vi "Func-엑셀 데이터를 그래프로 출력.vi"() -> ()   [LabVIEW 2015] (continued)
-4.925\n-18.3\t-18.32\t-4.927\n-18.3\t-18.32\t-4.934\n-18.3\t-18.32\t-4.936\n-18.3\t-18.32\t-4.944\n-18.3\t-18.32\t-4.95\n-18.3\t-18.32\t-4.957\n-18.3\t-18.32\t-4.965\n-18.3\t-18.32\t-4.972\n-18.3\t-18.32\t-4.976\n-18.3\t-18.32\t-4.977\n-18.3\t-18.32\t-4.984\n-18.3\t-18.32\t-4.99\n-18.3\t-18.32\t-4.997\n-18.3\t-18.32\t-5.002\n-18.3\t-18.32\t-5.007\n-18.3\t-18.32\t-5.013\n-18.3\t-18.32\t-5.02\n-18.3\t-18.32\t-5.023\n-18.3\t-18.32\t-5.024\n-18.3\t-18.32\t-5.031\n-18.3\t-18.32\t-5.036\n-18.3\t-18.32\t-5.041\n-18.3\t-18.32\t-5.047\n-18.3\t-18.32\t-5.053\n-18.3\t-18.32\t-5.061\n-18.3\t-18.32\t-5.069\n-18.3\t-18.32\t-5.075\n-18.3\t-18.32\t-5.08\n-18.3\t-18.32\t-5.085\n-18.3\t-18.32\t-5.091\n-18.3\t-18.32\t-5.092\n-18.3\t-18.32\t-5.099\n-18.3\t-18.32\t-5.105\n-18.3\t-18.32\t-5.109\n-18.3\t-18.32\t-5.117\n-18.3\t-18.32\t-5.122\n-18.3\t-18.32\t-5.13\n-18.3\t-18.32\t-5.134\n-18.3\t-18.32\t-5.137\n-18.3\t-18.32\t-5.142\n-18.3\t-18.32\t-5.146\n-18.3\t-18.32\t-5.15\n-18.3\t-18.32\t-5.152\n-18.3\t-18.32\t-5.16\n-18.3\t-18.32\t-5.164\n-18.3\t-18.32\t-5.166\n-18.3\t-18.32\t-5.177\n-18.3\t-18.32\t-5.183\n-18.3\t-18.32\t-5.187\n-18.3\t-18.32\t-5.19\n-18.3\t-18.31\t-5.196\n-18.3\t-18.31\t-5.202\n-18.3\t-18.31\t-5.205\n-18.3\t-18.31\t-5.209\n-18.3\t-18.31\t-5.214\n-18.3\t-18.31\t-5.219\n-18.3\t-18.31\t-5.223\n-18.3\t-18.31\t-5.225\n-18.3\t-18.31\t-5.231\n-18.3\t-18.31\t-5.235\n-18.3\t-18.31\t-5.24\n-18.3\t-18.31\t-5.25\n-18.3\t-18.31\t-5.254\n-18.3\t-18.31\t-5.262\n-18.3\t-18.31\t-5.269\n-18.3\t-18.31\t-5.274\n-18.3\t-18.31\t-5.279\n-18.3\t-18.31\t-5.28\n-18.3\t-18.31\t-5.287\n-18.3\t-18.31\t-5.291\n-18.3\t-18.31\t-5.298\n-18.3\t-18.31\t-5.302\n-18.3\t-18.31\t-5.305\n-18.3\t-18.31\t-5.312\n-18.3\t-18.31\t-5.312\n-18.3\t-18.31\t-5.318\n-18.3\t-18.31\t-5.323\n-18.3\t-18.31\t-5.328\n-18.3\t-18.31\t-5.334\n-18.3\t-18.31\t-5.346\n-18.3\t-18.31\t-5.353\n-18.3\t-18.31\t-5.354\n-18.3\t-18.31\t-5.36\n-18.3\t-18.31\t-5.363\n-18.3\t-18.31\t-5.363\n-18.3\t-18.31\t-5.367\n-18.3\t-18.31\t-5.372\n-18.3\t-18.31\t-5.378\n-18.3\t-18.31\t-5.384\n-18.3\t-18.31\t-5.391\n-18.3\t-18.31\t-5.398\n-18.3\t-18.31\t-5.402\n-18.3\t-18.31\t-5.407\n-18.3\t-18.31\t-5.411\n-18.3\t-18.31\t-5.416\n-18.3\t-18.31\t-5.418\n-18.3\t-18.31\t-5.423\n-18.3\t-18.31\t-5.427\n-18.3\t-18.31\t-5.43\n-18.3\t-18.31\t-5.437\n-18.3\t-18.31\t-5.442\n-18.3\t-18.31\t-5.447\n-18.3\t-18.31\t-5.451\n-18.3\t-18.31\t-5.459\n-18.3\t-18.31\t-5.461\n-18.3\t-18.31\t-5.463\n-18.3\t-18.31\t-5.469\n-18.3\t-18.31\t-5.473\n-18.3\t-18.31\t-5.48\n-18.3\t-18.31\t-5.485\n-18.3\t-18.31\t-5.489\n-18.3\t-18.31\t-5.495\n-18.3\t-18.31\t-5.504\n-18.3\t-18.31\t-5.509\n-18.3\t-18.31\t-5.511\n-18.3\t-18.31\t-5.516\n-18.3\t-18.31\t-5.519\n-18.3\t-18.29\t-5.52\n-18.3\t-18.29\t-5.523\n-18.3\t-18.29\t-5.529\n-18.3\t-18.29\t-5.533\n-18.3\t-18.29\t-5.54\n-18.3\t-18.29\t-5.546\n-18.3\t-18.29\t-5.555\n-18.3\t-18.29\t-5.56\n-18.3\t-18.29\t-5.563\n-18.3\t-18.29\t-5.564\n-18.3\t-18.29\t-5.571\n-18.3\t-18.29\t-5.575\n-18.3\t-18.29\t-5.576\n-18.3\t-18.29\t-5.582\n-18.3\t-18.29\t-5.584\n-18.3\t-18.29\t-5.591\n-18.3\t-18.29\t-5.593\n-18.3\t-18.29\t-5.596\n-18.3\t-18.29\t-5.602\n-18.3\t-18.29\t-5.606\n-18.3\t-18.29\t-5.61\n-18.3\t-18.29\t-5.614\n-18.3\t-18.29\t-5.62\n-18.3\t-18.29\t-5.626\n-18.3\t-18.29\t-5.63\n-18.3\t-18.29\t-5.639\n-18.3\t-18.29\t-5.645\n-18.3\t-18.29\t-5.647\n-18.3\t-18.29\t-5.654\n-18.3\t-18.29\t-5.658\n-18.3\t-18.29\t-5.66\n-18.3\t-18.29\t-5.661\n-18.3\t-18.29\t-5.664\n-18.3\t-18.29\t-5.668\n-18.3\t-18.29\t-5.673\n-18.3\t-18.29\t-5.675\n-18.3\t-18.29\t-5.684\n-18.3\t-18.29\t-5.69\n-18.3\t-18.29\t-5.689\n-18.3\t-18.29\t-5.695\n-18.3\t-18.29\t-5.702\n-18.3\t-18.29\t-5.705\n-18.3\t-18.29\t-5.703\n-18.3\t-18.29\t-5.709\n-18.3\t-18.29\t-5.719\n-18.3\t-18.29\t-5.721\n-18.3\t-18.29\t-5.722\n-18.3\t-18.29\t-5.723\n-18.3\t-18.29\t-5.729\n-18.3\t-18.29\t-5.734\n-18.3\t-18.29\t-5.732\n-18.3\t-18.29\t-5.736\n-18.3\t-18.29\t-5.745\n-18.3\t-18.29\t-5.754\n-18.3\t-18.29\t-5.759\n-18.3\t-18.29\t-5.765\n-18.3\t-18.29\t-5.773\n-18.3\t-18.29\t-5.778\n-18.3\t-18.29\t-5.782\n-18.3\t-18.29\t-5.786\n-18.3\t-18.29\t-5.791\n-18.3\t-18.29\t-5.791\n-18.3\t-18.29\t-5.796\n-18.3\t-18.29\t-5.798\n-18.3\t-18.29\t-5.803\n-18.3\t-18.29\t-5.804\n-18.3\t-18.29\t-5.811\n-18.3\t-18.29\t-5.816\n-18.3\t-18.29\t-5.82\n-18.3\t-18.29\t-5.826\n-18.3\t-18.29\t-5.829\n-18.3\t-18.29\t-5.836\n-18.3\t-18.29\t-5.838\n-18.3\t-18.29\t-5.845\n-18.3\t-18.29\t-5.843\n-18.3\t-18.29\t-5.85\n-18.3\t-18.29\t-5.855\n-18.3\t-18.29\t-5.859\n-18.3\t-18.29\t-5.861\n-18.3\t-18.29\t-5.863\n-18.3\t-18.29\t-5.871\n-18.3\t-18.29\t-5.876\n-18.3\t-18.29\t-5.878\n-18.3\t-18.29\t-5.882\n-18.3\t-18.29\t-5.889\n-18.3\t-18.29\t-5.89\n-18.3\t-18.29\t-5.892\n-18.3\t-18.29\t-5.895\n-18.3\t-18.29\t-5.9\n-18.3\t-18.29\t-5.903\n-18.3\t-18.29\t-5.912\n-18.3\t-18.29\t-5.915\n-18.3\t-18.29\t-5.92\n-18.3\t-18.29\t-5.925\n-18.3\t-18.29\t-5.929\n-18.3\t-18.29\t-5.931\n-18.3\t-18.29\t-5.933\n-18.3\t-18.29\t-5.938\n-18.3\t-18.29\t-5.941\n-18.3\t-18.29\t-5.945\n-18.3\t-18.29\t-5.945\n-18.3\t-18.29\t-5.949\n-18.3\t-18.29\t-5.955\n-18.3\t-18.29\t-5.958\n-18.3\t-18.29\t-5.965\n-18.3\t-18.29\t-5.97\n-18.3\t-18.29\t-5.977\n-18.3\t-18.29\t-5.981\n-18.3\t-18.29\t-5.983\n-18.3\t-18.29\t-5.987\n-18.3\t-18.29\t-5.988\n-18.3\t-18.29\t-5.993\n-18.3\t-18.29\t-5.998\n-18.3\t-18.29\t-5.999\n-18.3\t-18.29\t-6.005\n-18.3\t-18.29\t-6.01\n-18.3\t-18.29\t-6.015\n-18.3\t-18.29\t-6.019\n-18.3\t-18.29\t-6.019\n-18.3\t-18.29\t-6.025\n-18.3\t-18.29\t-6.029\n-18.3\t-18.29\t-6.032\n-18.3\t-18.29\t-6.034\n-18.3\t-18.29\t-6.038\n-18.3\t-18.29\t-6.043\n-18.3\t-18.29\t-6.046\n-18.3\t-18.29\t-6.048\n-18.3\t-18.29\t-6.052\n-18.3\t-18.29\t-6.052\n-18.3\t-18.29\t-6.055\n-18.3\t-18.29\t-6.059\n-18.3\t-18.29\t-6.065\n-18.3\t-18.29\t-6.074\n-18.3\t-18.29\t-6.078\n-18.3\t-18.29\t-6.083\n-18.3\t-18.29\t-6.087\n-18.3\t-18.29\t-6.091\n-18.3\t-18.29\t-6.092\n-18.3\t-18.29\t-6.095\n-18.3\t-18.29\t-6.095\n-18.3\t-18.29\t-6.101\n-18.3\t-18.28\t-6.105\n-18.3\t-18.28\t-6.108\n-18.3\t-18.28\t-6.111\n-18.3\t-18.28\t-6.115\n-18.3\t-18.28\t-6.124\n-18.3\t-18.28\t-6.123\n-18.3\t-18.28\t-6.131\n-18.3\t-18.28\t-6.135\n-18.3\t-18.28\t-6.139\n-18.3\t-18.28\t-6.148\n-18.3\t-18.28\t-6.147\n-18.3\t-18.28\t-6.148\n-18.3\t-18.28\t-6.151\n-18.3\t-18.28\t-6.155\n-18.3\t-18.28\t-6.156\n-18.3\t-18.28\t-6.155\n-18.3\t-18.28\t-6.162\n-18.3\t-18.28\t-6.172\n-18.3\t-18.28\t-6.177\n-18.3\t-18.28\t-6.177\n-18.3\t-18.28\t-6.183\n-18.3\t-18.28\t-6.187\n-18.3\t-18.28\t-6.19\n-18.3\t-18.28\t-6.189\n-18.3\t-18.28\t-6.196\n-18.3\t-18.28\t-6.199\n-18.3\t-18.28\t-6.2\n-18.3\t-18.28\t-6.202\n-18.3\t-18.28\t-6.204\n-18.3\t-18.28\t-6.208\n-18.3\t-18.28\t-6.211\n-18.3\t-18.29\t-6.214\n-18.3\t-18.29\t-6.219\n-18.3\t-18.29\t-6.228\n-18.3\t-18.29\t-6.232\n-18.3\t-18.29\t-6.235\n-18.3\t-18.29\t-6.237\n-18.3\t-18.29\t-6.243\n-18.3\t-18.29\t-6.247\n-18.3\t-18.29\t-6.248\n-18.3\t-18.29\t-6.248\n-18.3\t-18.29\t-6.252\n-18.3\t-18.29\t-6.257\n-18.3\t-18.29\t-6.256\n-18.3\t-18.29\t-6.259\n-18.3\t-18.29\t-6.263\n-18.3\t-18.29\t-6.268\n-18.3\t-18.29\t-6.271\n-18.3\t-18.29\t-6.276\n-18.3\t-18.29\t-6.282\n-18.3\t-18.29\t-6.281\n-18.3\t-18.29\t-6.283\n-18.3\t-18.29\t-6.286\n-18.3\t-18.29\t-6.289\n-18.3\t-18.29\t-6.296\n-18.3\t-18.29\t-6.295\n-18.3\t-18.29\t-6.3\n-18.3\t-18.29\t-6.305\n-18.3\t-18.29\t-6.309\n-18.3\t-18.29\t-6.312\n-18.3\t-18.29\t-6.312\n-18.3\t-18.29\t-6.315\n-18.3\t-18.29\t-6.319\n-18.3\t-18.29\t-6.324\n-18.3\t-18.29\t-6.325\n-18.3\t-18.29\t-6.328\n-18.3\t-18.29\t-6.332\n-18.3\t-18.29\t-6.338\n-18.3\t-18.29\t-6.341\n-18.3\t-18.29\t-6.345\n-18.3\t-18.29\t-6.351\n-18.3\t-18.29\t-6.358\n-18.3\t-18.29\t-6.361\n-18.3\t-18.29\t-6.365\n-18.3\t-18.29\t-6.368\n-18.3\t-18.29\t-6.371\n-18.3\t-18.29\t-6.371\n-18.3\t-18.29\t-6.373\n-18.3\t-18.29\t-6.375\n-18.3\t-18.29\t-6.375\n-18.3\t-18.29\t-6.378\n-18.3\t-18.29\t-6.385\n-18.3\t-18.29\t-6.388\n-18.3\t-18.29\t-6.391\n-18.3\t-18.29\t-6.394\n-18.3\t-18.29\t-6.4\n-18.3\t-18.29\t-6.405\n-18.3\t-18.29\t-6.407\n-18.3\t-18.29\t-6.409\n-18.3\t-18.29\t-6.417\n-18.3\t-18.29\t-6.417\n-18.3\t-18.29\t-6.418\n-18.3\t-18.29\t-6.421\n-18.3\t-18.29\t-6.421\n-18.3\t-18.29\t-6.426\n-18.3\t-18.29\t-6.427\n-18.3\t-18.29\t-6.432\n-18.3\t-18.29\t-6.432\n-18.3\t-18.29\t-6.434\n-18.3\t-18.31\t-6.439\n-18.3\t-18.31\t-6.439\n-18.3\t-18.31\t-6.446\n-18.3\t-18.31\t-6.448\n-18.3\t-18.31\t-6.454\n-18.3\t-18.31\t-6.457\n-18.3\t-18.31\t-6.459\n-18.3\t-18.31\t-6.464\n-18.3\t-18.31\t-6.465\n-18.3\t-18.31\t-6.468\n-18.3\t-18.31\t-6.473\n-18.3\t-18.31\t-6.478\n-18.3\t-18.31\t-6.48\n-18.3\t-18.31\t-6.481\n-18.3\t-18.31\t-6.489\n-18.3\t-18.31\t-6.493\n-18.3\t-18.31\t-6.494\n-18.3\t-18.31\t-6.498\n-18.3\t-18.31\t-6.502\n-18.3\t-18.31\t-6.507\n-18.3\t-18.31\t-6.509\n-18.3\t-18.31\t-6.51\n-18.3\t-18.31\t-6.514\n-18.3\t-18.31\t-6.518\n-18.3\t-18.31\t-6.523\n-18.3\t-18.31\t-6.526\n-18.3\t-18.31\t-6.531\n-18.3\t-18.31\t-6.532\n-18.3\t-18.31\t-6.534\n-18.3\t-18.31\t-6.537\n-18.3\t-18.31\t-6.536\n-18.3\t-18.31\t-6.537\n-18.3\t-18.31\t-6.541\n-18.3\t-18.31\t-6.545\n-18.3\t-18.31\t-6.547\n-18.3\t-18.31\t-6.554\n-18.3\t-18.31\t-6.56\n-18.3\t-18.31\t-6.561\n-18.3\t-18.31\t-6.565\n-18.3\t-18.31\t-6.568\n-18.3\t-18.31\t-6.572\n-18.3\t-18.31\t-6.575\n-18.3\t-18.31\t-6.579\n-18.3\t-18.31\t-6.584\n-18.3\t-18.31\t-6.586\n-18.3\t-18.31\t-6.588\n-18.3\t-18.31\t-6.589\n-18.3\t-18.31\t-6.591\n-18.3\t-18.31\t-6.595\n-18.3\t-18.31\t-6.599\n-18.3\t-18.31\t-6.601\n-18.3\t-18.31\t-6.601\n-18.3\t-18.31\t-6.605\n-18.3\t-18.31\t-6.607\n-18.3\t-18.31\t-6.606\n-18.3\t-18.31\t-6.609\n-18.3\t-18.31\t-6.611\n-18.3\t-18.31\t-6.614\n-18.3\t-18.31\t-6.618\n-18.3\t-18.31\t-6.622\n-18.3\t-18.31\t-6.624\n-18.3\t-18.31\t-6.627\n-18.3\t-18.31\t-6.629\n-18.3\t-18.31\t-6.633\n-18.3\t-18.31\t-6.634\n-18.3\t-18.31\t-6.634\n-18.3\t-18.31\t-6.639\n-18.3\t-18.31\t-6.645\n-18.3\t-18.31\t-6.648\n-18.3\t-18.31\t-6.65\n-18.3\t-18.31\t-6.654\n-18.3\t-18.31\t-6.655\n-18.3\t-18.31\t-6.655\n-18.3\t-18.31\t-6.657\n-18.3\t-18.31\t-6.66\n-18.3\t-18.31\t-6.664\n-18.3\t-18.31\t-6.666\n-18.3\t-18.31\t-6.673\n-18.3\t-18.31\t-6.676\n-18.3\t-18.31\t-6.677\n-18.3\t-18.31\t-6.679\n-18.3\t-18.31\t-6.684\n-18.3\t-18.31\t-6.689\n-18.3\t-18.31\t-6.689\n-18.3\t-18.31\t-6.69\n-18.3\t-18.31\t-6.698\n-18.3\t-18.31\t-6.704\n-18.3\t-18.31\t-6.703\n-18.3\t-18.31\t-6.705\n-18.3\t-18.31\t-6.709\n-18.3\t-18.31\t-6.71\n-18.3\t-18.31\t-6.711\n-18.3\t-18.31\t-6.708\n-18.3\t-18.31\t-6.711\n-18.3\t-18.31\t-6.713\n-18.3\t-18.31\t-6.716\n-18.3\t-18.31\t-6.721\n-18.3\t-18.31\t-6.728\n-18.3\t-18.31\t-6.734\n-18.3\t-18.31\t-6.738\n-18.3\t-18.31\t-6.743\n-18.3\t-18.31\t-6.746\n-18.3\t-18.31\t-6.751\n-18.3\t-18.31\t-6.751\n-18.3\t-18.31\t-6.75\n-18.3\t-18.31\t-6.749\n-18.3\t-18.31\t-6.748\n-18.3\t-18.31\t-6.75\n-18.3\t-18.31\t-6.75\n-18.3\t-18.31\t-6.752\n-18.3\t-18.31\t-6.755\n-18.3\t-18.31\t-6.759\n-18.3\t-18.31\t-6.769\n-18.3\t-18.31\t-6.774\n-18.3\t-18.31\t-6.78\n-18.3\t-18.31\t-6.782\n-18.3\t-18.31\t-6.784\n-18.3\t-18.31\t-6.787\n-18.3\t-18.31\t-6.787\n-18.3\t-18.31\t-6.787\n-18.3\t-18.31\t-6.787\n-18.3\t-18.31\t-6.792\n-18.3\t-18.31\t-6.796\n-18.3\t-18.31\t-6.802\n-18.3\t-18.31\t-6.804\n-18.3\t-18.31\t-6.804\n-18.3\t-18.31\t-6.809\n-18.3\t-18.31\t-6.81\n-18.3\t-18.31\t-6.809\n-18.3\t-18.31\t-6.809\n-18.3\t-18.31\t-6.814\n-18.3\t-18.31\t-6.818\n-18.3\t-18.31\t-6.818\n-18.3\t-18.31\t-6.822\n-18.3\t-18.31\t-6.826\n-18.3\t-18.31\t-6.827\n-18.3\t-18.31\t-6.831\n-18.3\t-18.31\t-6.83\n-18.3\t-18.31\t-6.835\n-18.3\t-18.31\t-6.839\n-18.3\t-18.31\t-6.84\n-18.3\t-18.31\t-6.843\n-18.3\t-18.31\t-6.845\n-18.3\t-18.31\t-6.851\n-18.3\t-18.31\t-6.851\n-18.3\t-18.31\t-6.854\n-18.3\t-18.31\t-6.858\n-18.3\t-18.31\t-6.863\n-18.3\t-18.31\t-6.867\n-18.3\t-18.31\t-6.867\n-18.3\t-18.31\t-6.87\n-18.3\t-18.31\t-6.876\n-18.3\t-18.31\t-6.879\n-18.3\t-18.31\t-6.879\n-18.3\t-18.31\t-6.882\n-18.3\t-18.31\t-6.888\n-18.3\t-18.31\t-6.89\n-18.3\t-18.31\t-6.892\n-18.3\t-18.31\t-6.891\n-18.3\t-18.31\t-6.895\n-18.3\t-18.31\t-6.896\n-18.3\t-18.31\t-6.895\n-18.3\t-18.31\t-6.896\n-18.3\t-18.31\t-6.898\n-18.3\t-18.31\t-6.901\n-18.3\t-18.31\t-6.902\n-18.3\t-18.31\t-6.907\n-18.3\t-18.31\t-6.91\n-18.3\t-18.31\t-6.915\n-18.3\t-18.31\t-6.92\n-18.3\t-18.31\t-6.924\n-18.3\t-18.31\t-6.927\n-18.3\t-18.31\t-6.933\n-18.3\t-18.31\t-6.938\n-18.3\t-18.31\t-6.941\n-18.3\t-18.31\t-6.942\n-18.3\t-18.31\t-6.947\n-18.3\t-18.31\t-6.951\n-18.3\t-18.31\t-6.95\n-18.3\t-18.31\t-6.951\n-18.3\t-18.31\t-6.954\n-18.3\t-18.31\t-6.959\n-18.3\t-18.31\t-6.958\n-18.3\t-18.31\t-6.957\n-18.3\t-18.31\t-6.961\n-18.3\t-18.31\t-6.966\n-18.3\t-18.31\t-6.968\n-18.3\t-18.31\t-6.968\n-18.3\t-18.32\t-6.969\n-18.3\t-18.32\t-6.972\n-18.3\t-18.32\t-6.974\n-18.3\t-18.32\t-6.974\n-18.3\t-18.32\t-6.973\n-18.3\t-18.32\t-6.973\n-18.3\t-18.32\t-6.977\n-18.3\t-18.32\t-6.979\n-18.3\t-18.32\t-6.984\n-18.3\t-18.32\t-6.988\n-18.3\t-18.32\t-6.991\n-18.3\t-18.32\t-6.998\n-18.3\t-18.32\t-6.999\n-18.3\t-18.32\t-7.002\n-18.3\t-18.32\t-7.003\n-18.3\t-18.32\t-7.005\n-18.3\t-18.32\t-7.007\n-18.3\t-18.32\t-7.009\n-18.3\t-18.32\t-7.012\n-18.3\t-18.32\t-7.016\n-18.3\t-18.32\t-7.02\n-18.3\t-18.32\t-7.02\n-18.3\t-18.32\t-7.023\n-18.3\t-18.32\t-7.027\n-18.3\t-18.32\t-7.028\n-18.3\t-18.32\t-7.029\n-18.3\t-18.32\t-7.027\n-18.3\t-18.32\t-7.029\n-18.3\t-18.32\t-7.03\n-18.3\t-18.32\t-7.028\n-18.3\t-18.32\t-7.03\n-18.3\t-18.32\t-7.032\n-18.3\t-18.31\t-7.039\n-18.3\t-18.31\t-7.041\n-18.3\t-18.31\t-7.047\n-18.3\t-18.31\t-7.053\n-18.3\t-18.31\t-7.056\n-18.3\t-18.31\t-7.062\n-18.3\t-18.31\t-7.062\n-18.3\t-18.31\t-7.062\n-18.3\t-18.31\t-7.064\n-18.3\t-18.31\t-7.067\n-18.3\t-18.31\t-7.068\n-18.3\t-18.31\t-7.067\n-18.3\t-18.31\t-7.071\n-18.3\t-18.31\t-7.073\n-18.3\t-18.31\t-7.075\n-18.3\t-18.31\t-7.077\n-18.3\t-18.32\t-7.081\n-18.3\t-18.31\t-7.083\n-18.3\t-18.31\t-7.084\n-18.3\t-18.31\t-7.086\n-18.3\t-18.31\t-7.088\n-18.3\t-18.31\t-7.091\n-18.3\t-18.31\t-7.089\n-18.3\t-18.31\t-7.095\n-18.3\t-18.31\t-7.096\n-18.3\t-18.31\t-7.097\n-18.3\t-18.31\t-7.102\n-18.3\t-18.32\t-7.105\n-18.3\t-18.32\t-7.109\n-18.3\t-18.31\t-7.107\n-18.3\t-18.32\t-7.11\n-18.3\t-18.31\t-7.114\n-18.3\t-18.31\t-7.118\n-18.3\t-18.31\t-7.118\n-18.3\t-18.31\t-7.121\n-18.3\t-18.31\t-7.13\n-18.3\t-18.31\t-7.134\n-18.3\t-18.31\t-7.137\n-18.3\t-18.31\t-7.138\n-18.3\t-18.31\t-7.139\n-18.3\t-18.31\t-7.138\n-18.3\t-18.31\t-7.136\n-18.3\t-18.31\t-7.139\n-18.3\t-18.31\t-7.14\n-18.3\t-18.31\t-7.143\n-18.3\t-18.31\t-7.146\n-18.3\t-18.31\t-7.148\n-18.3\t-18.31\t-7.155\n-18.3\t-18.31\t-7.157\n-18.3\t-18.31\t-7.156\n-18.3\t-18.31\t-7.16\n-18.3\t-18.31\t-7.161\n-18.3\t-18.31\t-7.164\n-18.3\t-18.31\t-7.166\n-18.3\t-18.31\t-7.168\n-18.3\t-18.31\t-7.17\n-18.3\t-18.31\t-7.171\n-18.3\t-18.31\t-7.175\n-18.3\t-18.32\t-7.178\n-18.3\t-18.31\t-7.182\n-18.3\t-18.32\t-7.181\n-18.3\t-18.32\t-7.186\n-18.3\t-18.32\t-7.187\n-18.3\t-18.32\t-7.191\n-18.3\t-18.32\t-7.189\n-18.3\t-18.32\t-7.191\n-18.3\t-18.31\t-7.193\n-18.3\t-18.31\t-7.193\n-18.3\t-18.31\t-7.197\n-18.3\t-18.31\t-7.2\n-18.3\t-18.31\t-7.209\n-18.3\t-18.31\t-7.213\n-18.3\t-18.32\t-7.214\n-18.3\t-18.32\t-7.215\n-18.3\t-18.32\t-7.213\n-18.3\t-18.32\t-7.214\n-18.3\t-18.32\t-7.213\n-18.3\t-18.31\t-7.214\n-18.3\t-18.31\t-7.218\n-18.3\t-18.31\t-7.222\n-18.3\t-18.31\t-7.231\n-18.3\t-18.31\t-7.23\n-18.3\t-18.31\t-7.23\n-18.3\t-18.31\t-7.234\n-18.3\t-18.31\t-7.234\n-18.3\t-18.31\t-7.234\n-18.3\t-18.31\t-7.236\n-18.3\t-18.31\t-7.241\n-18.3\t-18.31\t-7.244\n-18.3\t-18.31\t-7.243\n-18.3\t-18.31\t-7.246\n-18.3\t-18.31\t-7.249\n-18.3\t-18.31\t-7.25\n-18.3\t-18.31\t-7.254\n-18.3\t-18.31\t-7.255\n-18.3\t-18.31\t-7.257\n-18.3\t-18.31\t-7.262\n-18.3\t-18.31\t-7.263\n-18.3\t-18.31\t-7.262\n-18.3\t-18.31\t-7.264\n-18.3\t-18.31\t-7.266\n-18.3\t-18.31\t-7.27\n-18.3\t-18.31\t-7.267\n-18.3\t-18.31\t-7.271\n-18.3\t-18.31\t-7.275\n-18.3\t-18.31\t-7.275\n-18.3\t-18.31\t-7.277\n-18.3\t-18.31\t-7.28\n-18.3\t-18.31\t-7.284\n-18.3\t-18.31\t-7.287\n-18.3\t-18.31\t-7.289\n-18.3\t-18.31\t-7.292\n-18.3\t-18.31\t-7.295\n-18.3\t-18.31\t-7.297\n-18.3\t-18.31\t-7.299\n-18.3\t-18.31\t-7.3\n-18.3\t-18.31\t-7.304\n-18.3\t-18.31\t-7.305\n-18.3\t-18.31\t-7.309\n-18.3\t-18.31\t-7.312\n-18.3\t-18.31\t-7.313\n-18.3\t-18.31\t-7.316\n-18.3\t-18.31\t-7.318\n-18.3\t-18.31\t-7.321\n-18.3\t-18.31\t-7.321\n-18.3\t-18.31\t-7.321\n-18.3\t-18.31\t-7.323\n-18.3\t-18.31\t-7.323\n-18.3\t-18.31\t-7.328\n-18.3\t-18.31\t-7.328\n-18.3\t-18.31\t-7.329\n-18.3\t-18.31\t-7.333\n-18.3\t-18.31\t-7.337\n-18.3\t-18.31\t-7.341\n-18.3\t-18.31\t-7.343\n-18.3\t-18.31\t-7.344\n-18.3\t-18.31\t-7.347\n-18.3\t-18.31\t-7.343\n-18.3\t-18.31\t-7.341\n-18.3\t-18.31\t-7.341\n-18.3\t-18.31\t-7.342\n-18.3\t-18.31\t-7.343\n-18.3\t-18.31\t-7.344\n-18.3\t-18.31\t-7.352\n-18.3\t-18.31\t-7.36\n-18.3\t-18.31\t-7.359\n-18.3\t-18.31\t-7.361\n-18.3\t-18.31\t-7.366\n-18.3\t-18.31\t-7.368\n-18.3\t-18.31\t-7.37\n-18.3\t-18.31\t-7.369\n-18.3\t-18.31\t-7.377\n-18.3\t-18.31\t-7.379\n-18.3\t-18.31\t-7.379\n-18.3\t-18.31\t-7.381\n-18.3\t-18.31\t-7.385\n-18.3\t-18.31\t-7.384\n-18.3\t-18.31\t-7.385\n-18.3\t-18.31\t-7.385\n-18.3\t-18.31\t-7.384\n-18.3\t-18.31\t-7.385\n-18.3\t-18.31\t-7.385\n-18.3\t-18.31\t-7.389\n-18.3\t-18.31\t-7.391\n-18.3\t-18.31\t-7.393\n-18.3\t-18.31\t-7.396\n-18.3\t-18.31\t-7.396\n-18.3\t-18.31\t-7.394\n-18.3\t-18.31\t-7.395\n-18.3\t-18.31\t-7.398\n-18.3\t-18.31\t-7.399\n-18.3\t-18.31\t-7.4\n-18.3\t-18.31\t-7.404\n-18.3\t-18.31\t-7.409\n-18.3\t-18.31\t-7.409\n-18.3\t-18.31\t-7.412\n-18.3\t-18.31\t-7.416\n-18.3\t-18.31\t-7.42\n-18.3\t-18.31\t-7.421\n-18.3\t-18.31\t-7.424\n-18.3\t-18.31\t-7.425\n-18.3\t-18.31\t-7.423\n-18.3\t-18.31\t-7.426\n-18.3\t-18.31\t-7.424\n-18.3\t-18.31\t-7.426\n-18.3\t-18.31\t-7.426\n-18.3\t-18.31\t-7.429\n-18.3\t-18.31\t-7.434\n-18.3\t-18.31\t-7.434\n-18.3\t-18.31\t-7.438\n-18.3\t-18.31\t-7.444\n-18.3\t-18.31\t-7.446\n-18.3\t-18.31\t-7.451\n-18.3\t-18.31\t-7.452\n-18.3\t-18.31\t-7.456\n-18.3\t-18.31\t-7.459\n-18.3\t-18.31\t-7.459\n-18.3\t-18.31\t-7.462\n-18.3\t-18.31\t-7.462\n-18.3\t-18.31\t-7.464\n-18.3\t-18.31\t-7.466\n-18.3\t-18.31\t-7.469\n-18.3\t-18.31\t-7.473\n-18.3\t-18.31\t-7.475\n-18.3\t-18.31\t-7.475\n-18.3\t-18.31\t-7.479\n-18.3\t-18.31\t-7.479\n-18.3\t-18.31\t-7.478\n-18.3\t-18.31\t-7.48\n-18.3\t-18.31\t-7.48\n-18.3\t-18.31\t-7.483\n-18.3\t-18.31\t-7.481\n-18.3\t-18.31\t-7.486\n-18.3\t-18.31\t-7.488\n-18.3\t-18.31\t-7.488\n-18.3\t-18.31\t-7.492\n-18.3\t-18.31\t-7.491\n-18.3\t-18.31\t-7.495\n-18.3\t-18.31\t-7.493\n-18.3\t-18.31\t-7.493\n-18.3\t-18.31\t-7.498\n-18.3\t-18.31\t-7.497\n-18.3\t-18.31\t-7.502\n-18.3\t-18.31\t-7.505\n-18.3\t-18.31\t-7.51\n-18.3\t-18.31\t-7.512\n-18.3\t-18.31\t-7.509\n-18.3\t-18.31\t-7.514\n-18.3\t-18.31\t-7.516\n-18.3\t-18.31\t-7.516\n-18.3\t-18.31\t-7.514\n-18.3\t-18.31\t-7.517\n-18.3\t-18.31\t-7.519\n-18.3\t-18.31\t-7.52\n-18.3\t-18.31\t-7.52\n-18.3\t-18.31\t-7.523\n-18.3\t-18.31\t-7.528\n-18.3\t-18.31\t-7.53\n-18.3\t-18.31\t-7.538\n-18.3\t-18.31\t-7.539\n-18.3\t-18.31\t-7.539\n-18.3\t-18.31\t-7.546\n-18.3\t-18.31\t-7.547\n-18.3\t-18.31\t-7.545\n-18.3\t-18.31\t-7.545\n-18.3\t-18.31\t-7.547\n-18.3\t-18.31\t-7.552\n-18.3\t-18.31\t-7.548\n-18.3\t-18.31\t-7.547\n-18.3\t-18.31\t-7.552\n-18.3\t-18.31\t-7.555\n-18.3\t-18.31\t-7.555\n-18.3\t-18.31\t-7.557\n-18.3\t-18.31\t-7.559\n-18.3\t-18.31\t-7.563\n-18.3\t-18.31\t-7.562\n-18.3\t-18.31\t-7.561\n-18.3\t-18.31\t-7.564\n-18.3\t-18.31\t-7.563\n-18.3\t-18.31\t-7.568\n-18.3\t-18.31\t-7.569\n-18.3\t-18.31\t-7.573\n-18.3\t-18.31\t-7.579\n-18.3\t-18.31\t-7.58\n-18.3\t-18.31\t-7.587\n-18.3\t-18.31\t-7.586\n-18.3\t-18.31\t-7.589\n-18.3\t-18.31\t-7.589\n-18.3\t-18.31\t-7.588\n-18.3\t-18.31\t-7.589\n-18.3\t-18.31\t-7.588\n-18.3\t-18.31\t-7.592\n-18.3\t-18.31\t-7.591\n-18.3\t-18.31\t-7.593\n-18.3\t-18.31\t-7.598\n-18.3\t-18.31\t-7.598\n-18.3\t-18.31\t-7.6\n-18.3\t-18.31\t-7.603\n-18.3\t-18.31\t-7.607\n-18.3\t-18.31\t-7.61\n-18.3\t-18.31\t-7.608\n-18.3\t-18.31\t-7.613\n-18.3\t-18.31\t-7.613\n-18.3\t-18.31\t-7.612\n-18.3\t-18.31\t-7.609\n-18.3\t-18.31\t-7.612\n-18.3\t-18.31\t-7.617\n-18.3\t-18.31\t-7.617\n-18.3\t-18.31\t-7.618\n-18.3\t-18.31\t-7.624\n-18.3\t-18.31\t-7.629\n-18.3\t-18.31\t-7.629\n-18.3\t-18.31\t-7.628\n-18.3\t-18.31\t-7.628\n-18.3\t-18.31\t-7.632\n-18.3\t-18.31\t-7.632\n-18.3\t
